vi "VIQA Initialize.vi"(8 "error in (no error)":errorcluster, 9 "Filter":T1, 10 "Project Tree":refnum<vi>, 11 "Project (*.lvproj)":path) -> (0 "error out":errorcluster, 2 "My Computer":refnum<vi>, 3 "Project":refnum<vi>, 5 "App Ref":refnum<vi>)   [LabVIEW 2018, in "VI Quality.lvlib"]
doc: "This VI opens a LabVIEW project and initializes the project items tree"
uses:
  VI Quality.lvlib
  Controls/VIQA Filter.ctl
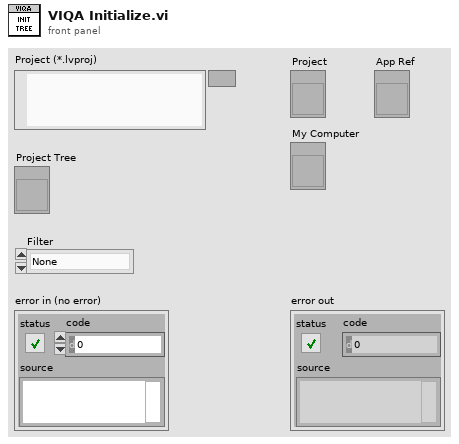
[diagram p1: front panel]
types:
  T1 = typedef "VI Quality.lvlib/VIQA Filter.ctl" = enum16{"None", "No Description"}
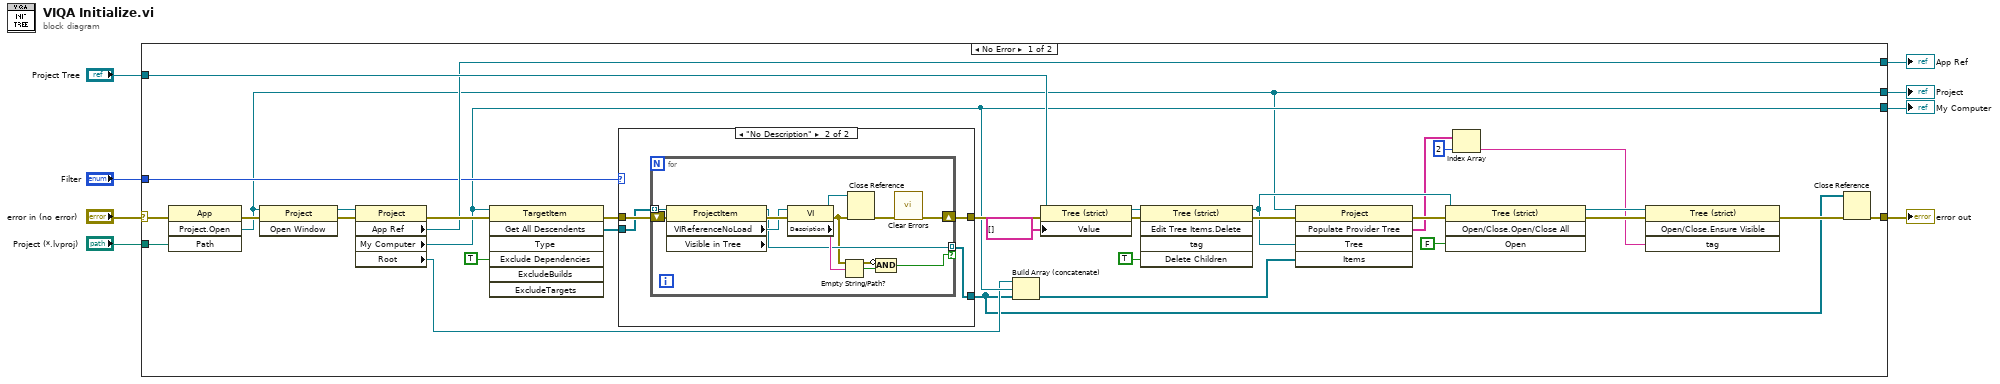
[diagram p0: block diagram]
diagram:
  n1 = case shown="No Error" "error in (no error)" {
    selector: "error in (no error)" -> [w31 w60]
    tunnel: "Project (*.lvproj)" -> [w41 _]
    tunnel: [w11 _] -> w7
    tunnel: [w20 _] -> w6
    tunnel: "Project Tree" -> [w28 _]
    tunnel: [w30 w60] -> w3
    tunnel: [w25 _] -> w2
    tunnel: "Filter" -> [w22 _]
    frame No Error {
      n2 = invoke class="App" method="Project.Open"(error in=w31, "Path"=w41) -> (error out=w39:errorcluster, "Project:Open"=w11:refnum<vi>)  [unwired: 2 in, 2 out]
      n3 = invoke class="Project" method="Open Window"(reference=w11, error in=w39) -> (reference out=w10:refnum<vi>, error out=w12:errorcluster)  [unwired: 1 in, 1 out]
      n4 = property class="Project"(reference=w10, error in=w12) -> (error out=w38:errorcluster, "App Ref"=w25:refnum<vi>, "My Computer"=w20:refnum<vi>, "Root"=w18:refnum<vi>)  [unwired: 1 out]
      n5 = invoke class="TargetItem" method="Get All Descendents"(reference=w20, error in=w38, "Exclude Dependencies"=TRUE ("ExcludeDependencies")) -> (error out=w36:errorcluster, "All Descendents"=w23:refnum<vi>[])  [unwired: 4 in, 5 out]
      n6 = case shown="\"No Description\"" w22 {
        tunnel: w36 -> [w42 w47]
        tunnel: [w42 w46] -> w24
        tunnel: w23 -> [w43 w45]
        tunnel: [w43 w44] -> w9
        frame "None", Default {
        }
        frame "No Description" {
          n7 = for {
            tunnel: w45 -> [w57] mode=indexing
            shift-right: [w51] -> w46
            shift-left: w47 -> [w59]
            tunnel: [w54] -> w44 mode=indexing if=w48
            n8 = property class="ProjectItem" props=["VIReferenceNoLoad", "Visible in Tree"](reference=w57, error in=w59) -> (reference out=w54:refnum<vi>, error out=w58:errorcluster, "VIReferenceNoLoad"=w56:refnum<vi>)  [unwired: 1 out]
            n9 = property class="VI"(reference=w56, error in=w58) -> (reference out=w52:refnum<vi>, error out=w49:errorcluster, "Description"=w55:string)
            n10 = Empty String/Path?(string/path=w55) -> (empty?=w50:bool)
            n11 = Close Reference(reference=w52, error in (no error)=w49) -> (error out=w53:errorcluster)
            n12 = Compound Arithmetic op=AND(invert w49, w50) -> (w48:bool)
            n13 = call <vilib>:"Clear Errors.vi"("error in (no error)"=w53) -> ("error out"=w51:errorcluster)  [unwired: 5 in, 1 out]
          }
        }
      }
      n14 = Build Array (concatenate)(w18, w20, w9) -> (w19:refnum<vi>[])
      n15 = property class="Tree (strict)"(reference=w28, error in=w24, "Value"=string[] []) -> (reference out=w27:refnum<vi>, error out=w29:errorcluster)
      n16 = invoke class="Tree (strict)" method="Edit Tree Items.Delete"(reference=w27, error in=w29, "Delete Children"=TRUE ("Delete Children?")) -> (reference out=w21:refnum<vi>, error out=w35:errorcluster)  [unwired: 2 in, 3 out]
      n17 = invoke class="Project" method="Populate Provider Tree"(reference=w11, error in=w35, "Tree"=w21, "Items"=w19) -> (error out=w40:errorcluster, "Populate Provider Tree"=w15:string[])  [unwired: 1 in, 3 out]
      n18 = invoke class="Tree (strict)" method="Open/Close.Open/Close All"(reference=w21, error in=w40, "Open"=FALSE ("Open?")) -> (reference out=w16:refnum<vi>, error out=w32:errorcluster)  [unwired: 1 in, 2 out]
      n19 = Index Array(array=w15, index=2) -> (element=w13:string)
      n20 = invoke class="Tree (strict)" method="Open/Close.Ensure Visible"(reference=w16, error in=w32, "tag"=w13) -> (error out=w17:errorcluster)  [unwired: 1 in, 3 out]
      n21 = Close Reference(reference=w9, error in (no error)=w17) -> (error out=w30:errorcluster)
    }
    frame Error {
    }
  }
  "error out" <- w3
  "Project" <- w7
  "My Computer" <- w6
  "App Ref" <- w2
